vi "The Plant and its parameters (v. 2020).vi"() -> ()   [LabVIEW 2019]
panel:
  out "Plant Output":dbl(slide) scale=0.0..100.0
  in  "stop":bool
  in  "Plant Parameters":T1
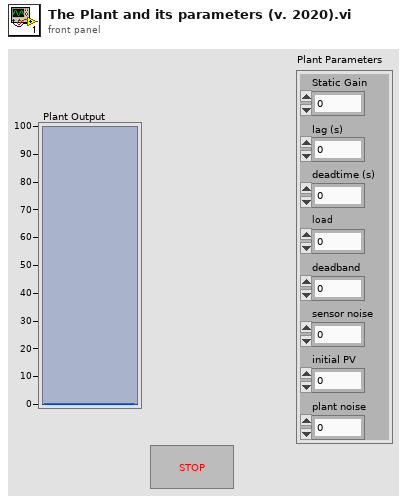
[diagram p1: front panel]
types:
  T1 = cluster{"Static Gain":dbl, "lag (s)":dbl, "deadtime (s)":dbl, "load":dbl, "deadband":dbl, "sensor noise":dbl, "initial PV":dbl, "plant noise":dbl}
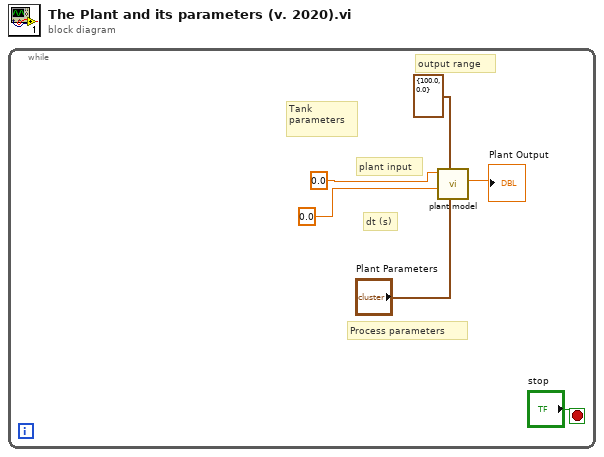
[diagram p0: block diagram]
diagram:
  n1 = while {
    stop <- "stop" stop-if-true
    # "dt (s)"
    # "plant input"
    # "Tank \nparameters"
    # "Process parameters"
    # "output range"
    n2 = call "plant model.vi"("process parameters"="Plant Parameters", "output saturation range"=cluster{"output high":dbl, "output low":dbl} {"output high"=100.0, "output low"=0.0}, "dt (s)"=0.0, "Plant Input"=0.0) -> ("Plant Output"=→"Plant Output":dbl)  [unwired: 7 in]
  }
